vi "Batch Retrieve Cartesian Offsets.vi"(6 "error in (no error)":errorcluster, 7 "Force Offsets":T1[](array[typedef]), 8 "Displacement Offsets":T1[](array[typedef]), 9 "Force Tag":string) -> (0 "error out":errorcluster, 2 "Offsets":dbl[][](array[numeric]))   [LabVIEW 2009]
uses:
  Global Data/Dataset Transaction Id.ctl
  Global Data/Dataset Source.ctl
  Global Data/Dataset Type.ctl
  Apps/Yes No Button.ctl
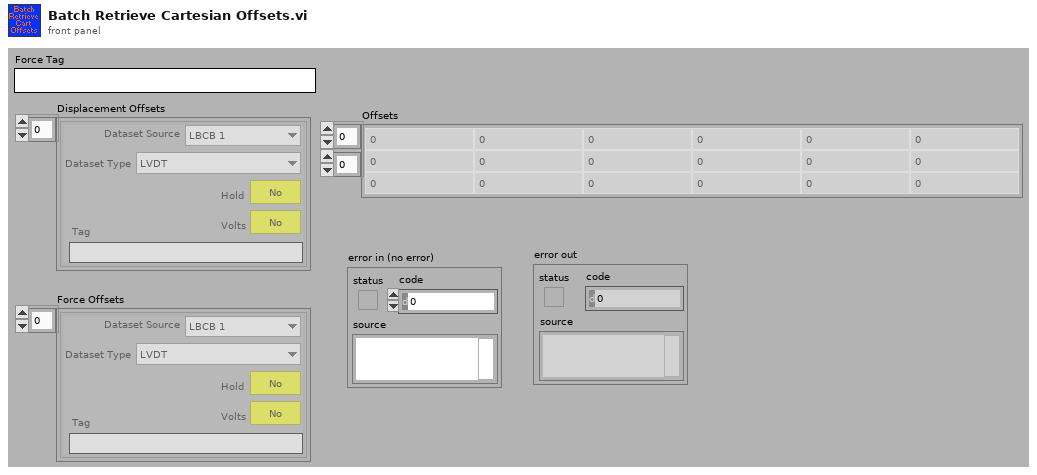
[diagram p1: front panel]
types:
  T1 = typedef "Dataset Transaction Id.ctl" = cluster{"Dataset Source":T2, "Dataset Type":T3, "Hold":T4, "Volts":T4, "Tag":string}
  T2 = typedef "Dataset Source.ctl" = enum16{"LBCB 1", "LBCB 2", "Combined", "External Sensors"}
  T3 = typedef "Dataset Type.ctl" = enum16{"LVDT", "Load Cell", "Actuator Command", "Servo Error", "Displacement Command", "Displacement", "Force"}
  T4 = typedef "Yes No Button.ctl" = bool
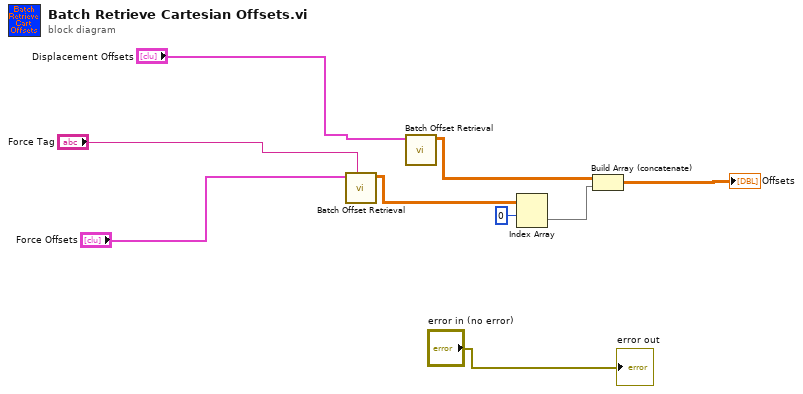
[diagram p0: block diagram]
diagram:
  n1 = call "Batch Offset Retrieval.vi"("Tag"="Force Tag", "Transactions"="Force Offsets") -> ("Data"=w4:dbl[][])  [unwired: 8 in, 1 out]
  n2 = call "Batch Offset Retrieval.vi"("Transactions"="Displacement Offsets") -> ("Data"=w2:dbl[][])  [unwired: 9 in, 1 out]
  n3 = Index Array(array=w4, index (row)=0) -> (element=w1:dbl[])  [unwired: 1 in]
  n4 = Build Array (concatenate)(w2, w1) -> (→"Offsets":dbl[][])
  "error out" <- "error in (no error)"
